vi "get lvdt value_keyence DL-EP1.vi"(7 "Preset Command":dbl, 8 "error in":errorcluster, 9 "update preset":bool, 10 "Instance ID in  (LVDT Amplifier Index [1..n])":u32, 11 "Network Path":string) -> (0 "error out":errorcluster, 2 "Zero-Offset":dbl, 3 "PV":dbl)   [LabVIEW 2018]
uses:
  <vilib>/ethernetip/ethernetip.lvlib
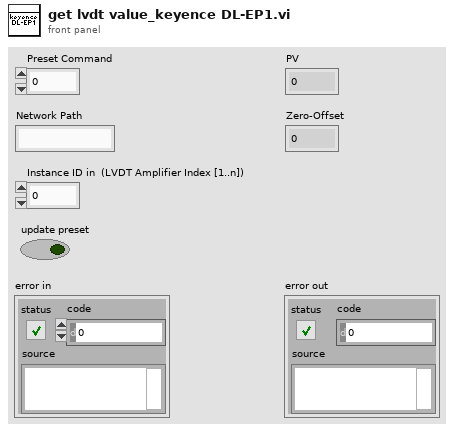
[diagram p1: front panel]
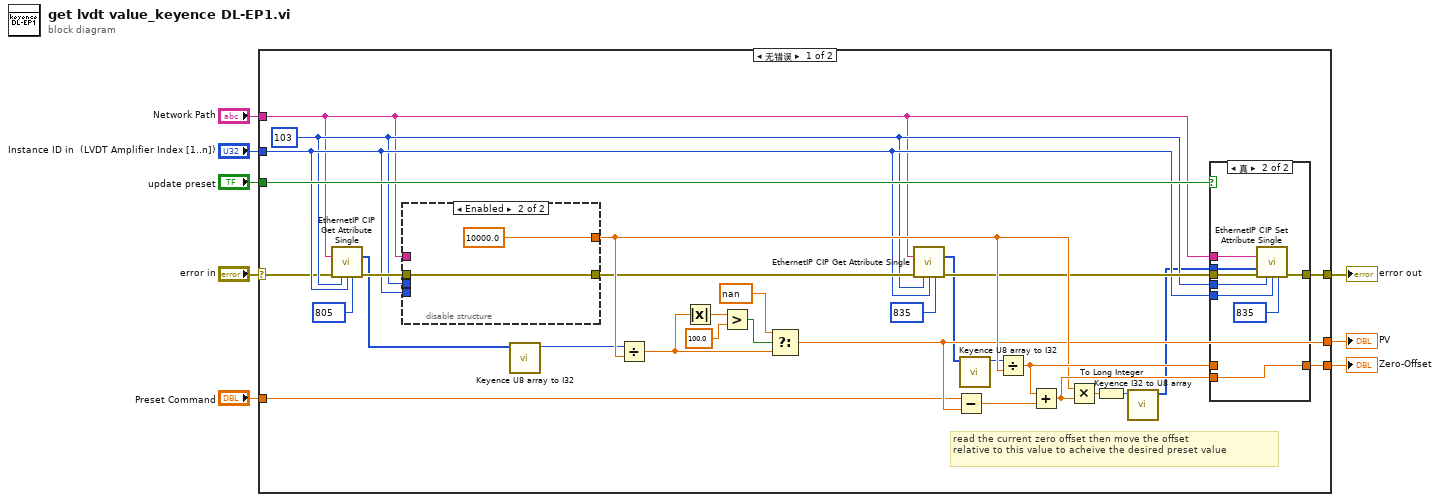
[diagram p0: block diagram]
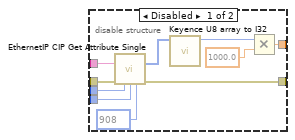
[diagram p2: hidden frame]
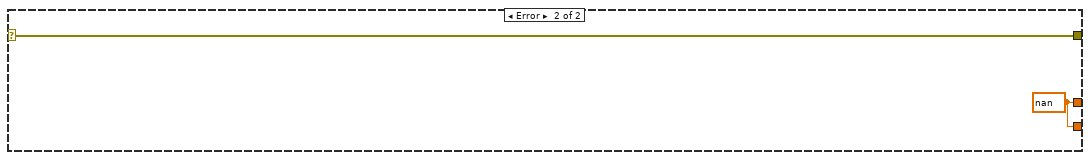
[diagram p4: hidden frame]
diagram:
  n1 = case shown="无错误" "error in" {
    selector: "error in" -> [w9 w62]
    tunnel: [w35 w61] -> w8
    tunnel: [w34 w62] -> w7
    tunnel: [w28 w61] -> w6
    tunnel: "update preset" -> [w23 _]
    tunnel: "Preset Command" -> [w21 _]
    tunnel: "Instance ID in  (LVDT Amplifier Index [1..n])" -> [w17 _]
    tunnel: "Network Path" -> [w15 _]
    frame No Error {
      w16 = u32 103 ("Instance ID in")
      # "read the current zero offset then move the offset\nrelative to this value to acheive the desired preset value"
      n2 = call <vilib>:"EthernetIP CIP Get Attribute Single.vi"("Network Path"=w15, "error in"=w9, "Class"=w16, "Instance"=w17, "Attribute"=u32 805 ("Instance ID in")) -> ("Data"=w11:u8[], "error out"=w30:errorcluster)  [unwired: 8 in, 1 out]
      n3 = disable-structure shown="Enabled" {
        disable-tunnel: w15 -> [w46 _]
        disable-tunnel: w16 -> [w45 _]
        disable-tunnel: w17 -> [w44 _]
        disable-tunnel: [w43 10000.0] -> w33
        disable-tunnel: w30 -> [w40 w49]
        disable-tunnel: [w39 w49] -> w31
        frame Disabled {
          n4 = call <vilib>:"EthernetIP CIP Get Attribute Single.vi"("Network Path"=w46, "error in"=w40, "Class"=w45, "Instance"=w44, "Attribute"=u32 908 ("Instance ID in")) -> ("Data"=w47:u8[], "error out"=w39:errorcluster)  [unwired: 8 in, 1 out]
          n5 = call "Keyence U8 array to I32.vi"("U8 Array"=w47) -> ("I32"=w42:i32)  [unwired: 10 in]
          n6 = Multiply(x=w42, y=1000.0) -> (x*y=w43:dbl)
        }
        frame Enabled {
        }
      }
      n7 = call "Keyence U8 array to I32.vi"("U8 Array"=w11) -> ("I32"=w14:i32)  [unwired: 10 in]
      n8 = Divide(x=w14, y=w33) -> (x/y=w27:dbl)
      n9 = Absolute Value(x=w27) -> (abs(x)=w25:dbl)
      n10 = Greater?(x=w25, y=100.0) -> (0:w26:bool)
      n11 = Select(t=nan, s=w26, f=w27) -> (s? t:f=w28:dbl)
      n12 = call <vilib>:"EthernetIP CIP Get Attribute Single.vi"("Network Path"=w15, "error in"=w31, "Class"=w16, "Instance"=w17, "Attribute"=u32 835 ("Instance ID in")) -> ("Data"=w19:u8[], "error out"=w32:errorcluster)  [unwired: 8 in, 1 out]
      n13 = Subtract(x=w21, y=w28) -> (x-y=w22:dbl)
      n14 = call "Keyence U8 array to I32.vi"("U8 Array"=w19) -> ("I32"=w20:i32)  [unwired: 10 in]
      n15 = Divide(x=w20, y=w33) -> (x/y=w36:dbl)
      n16 = Add(x=w36, y=w22) -> (x+y=w38:dbl)
      n17 = Multiply(x=w33, y=w38) -> (x*y=w37:dbl)
      n18 = To Long Integer(number=w37) -> (32bit integer=w12:i32)
      n19 = call "Keyence I32 to U8 array.vi"("Numeric"=w12) -> ("Array"=w13:u8[])  [unwired: 10 in]
      n20 = case shown="真" w23 {
        tunnel: w13 -> [_ w60]
        tunnel: w15 -> [_ w59]
        tunnel: w16 -> [_ w58]
        tunnel: w17 -> [_ w57]
        tunnel: w32 -> [w52 w55]
        tunnel: [w52 w54] -> w34
        tunnel: [w51 w53] -> w35
        tunnel: w36 -> [w51 _]
        tunnel: w38 -> [_ w53]
        frame False {
        }
        frame True {
          n21 = call <vilib>:"EthernetIP CIP Set Attribute Single.vi"("Network Path"=w59, "Data"=w60, "error in"=w55, "Class"=w58, "Instance"=w57, "Attribute"=u32 835 ("Instance ID in")) -> ("error out"=w54:errorcluster)  [unwired: 8 in, 1 out]
        }
      }
    }
    frame Error {
      w61 = nan ("t")
    }
  }
  "Zero-Offset" <- w8
  "error out" <- w7
  "PV" <- w6
